vi "Mathtext2002.vi"   [LabVIEW 2013]
uses:
  <vilib>/Heliosphere Research LLC/Advanced Plotting Toolkit/Advanced Plotting Toolkit.lvlib
types:
  T1 = typedef "Advanced Plotting Toolkit.lvlib/PlotID.ctl" = i32
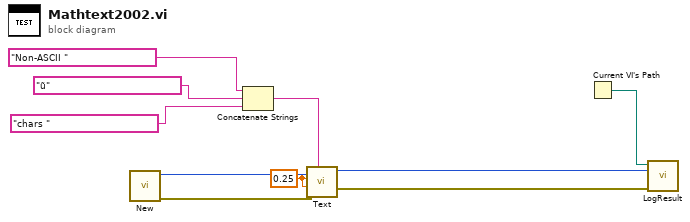
[diagram p0: block diagram]
diagram:
  w9 = 0.25 ("X Position")
  n1 = call <vilib>:"New.vi"() -> ("error out"=w7:errorcluster, "Plot ID"=w8:T1)  [unwired: 10 in]
  n2 = Concatenate Strings("Non-ASCII " ("Text"), "ũ" ("Text"), "chars " ("Text")) -> (w1:string)
  n3 = call <vilib>:"Text.vi"("Text"=w1, "error in (no error)"=w7, "Y Position"=w9, "X Position"=w9, "Plot ID"=w8) -> ("error out"=w5:errorcluster, "Plot ID Out"=w6:T1)  [unwired: 5 in]
  n4 = Current VI's Path() -> (path=w10:path)
  n5 = call "LogResult.vi"("Test Result"=w5, "Test Artifact"=w6, "VI Path"=w10) -> ()  [unwired: 9 in]
